vi "Extract Ring Text (SubVI).vi"(11 "Spreadsheet String":string[](array[string])) -> (3 "Output String":string[](array[string]))   [LabVIEW 2020]
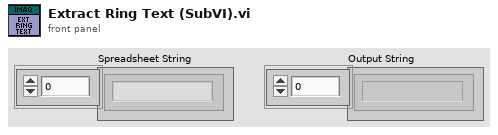
[diagram p1: front panel]
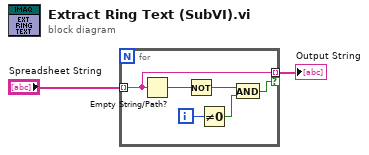
[diagram p0: block diagram]
diagram:
  n1 = for {
    tunnel: "Spreadsheet String" -> [w5] mode=indexing
    tunnel: [w5] -> w2 mode=indexing if=w4
    i -> [w8]
    n2 = Empty String/Path?(string/path=w5) -> (empty?=w7:bool)
    n3 = Not(x=w7) -> (.not. x?=w3:bool)
    n4 = Not Equal To 0?(x=w8) -> (x != 0?=w6:bool)
    n5 = And(x=w3, y=w6) -> (x .and. y?=w4:bool)
  }
  "Output String" <- w2
